vi "DLP232PC_Connection(SubVI).vi"(8 "error in (no error)":errorcluster, 11 "String":string) -> (0 "error out":errorcluster, 2 "Boolean":bool, 3 "VISA Refnum out":refnum<visa-resource-name>)   [LabVIEW 2022 SP3]
uses:
  <vilib>/Instr/_visa.llb/VISA Configure Serial Port (Instr).vi
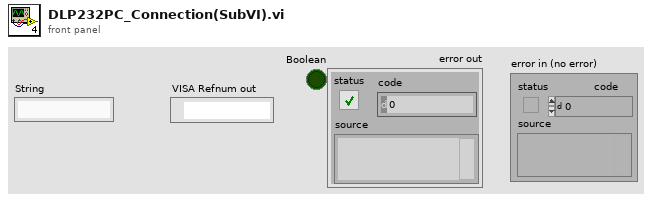
[diagram p1: front panel]
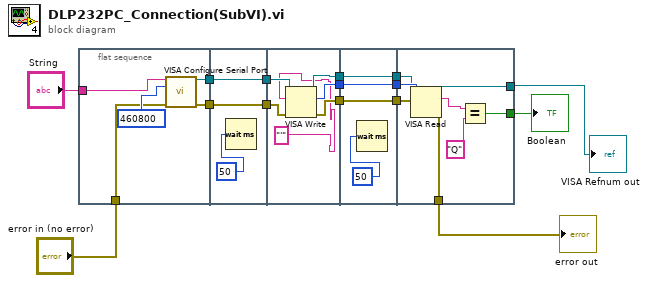
[diagram p0: block diagram]
diagram:
  n1 = flat-sequence {
    tunnel: [w19] -> w15
    tunnel: [w18] -> w14
    tunnel: "String" -> [w17]
    tunnel: "error in (no error)" -> [w16]
    tunnel: w15 -> [w23]
    tunnel: w14 -> [w22]
    tunnel: [w23] -> w13
    tunnel: [w22] -> w12
    tunnel: w13 -> [w28]
    tunnel: w12 -> [w29]
    tunnel: [w27] -> w11
    tunnel: [w26] -> w10
    tunnel: [w25] -> w9
    tunnel: w11 -> [w33]
    tunnel: w10 -> [w32]
    tunnel: w9 -> [w31]
    tunnel: [w33] -> w8
    tunnel: [w32] -> w7
    tunnel: [w31] -> w6
    tunnel: w8 -> [w39]
    tunnel: w7 -> [w38]
    tunnel: w6 -> [w37]
    tunnel: [w36] -> w3
    tunnel: [w35] -> w4
    tunnel: [w34] -> w2
    frame #0 {
      n2 = call-poly "VISA Configure Serial Port"("VISA resource name"=w17, "baud rate (9600)"=u32 460800, "error in (no error)"=w16) -> ("VISA resource name out"=w19:refnum<visa-resource-name>, "error out"=w18:errorcluster)  [unwired: 11 in]
    }
    frame #1 {
      n3 = Wait (ms)(milliseconds to wait=u32 50) -> ()  [unwired: 1 out]
    }
    frame #2 {
      n4 = VISA Write(VISA resource name=w28, write buffer="'" ("string"), error in (no error)=w29) -> (VISA resource name out=w25:refnum<visa-resource-name>, return count=w26:u32, error out=w27:errorcluster)
    }
    frame #3 {
      n5 = Wait (ms)(milliseconds to wait=u32 50) -> ()  [unwired: 1 out]
    }
    frame #4 {
      n6 = VISA Read(VISA resource name=w37, byte count=w38, error in (no error)=w39) -> (VISA resource name out=w35:refnum<visa-resource-name>, read buffer=w41:string, error out=w34:errorcluster)  [unwired: 1 out]
      n7 = Equal?(x=w41, y="Q") -> (x = y?=w36:bool)
    }
  }
  "VISA Refnum out" <- w4
  "Boolean" <- w3
  "error out" <- w2
